vi "Get Connection from Statement.vi"(8 "error in (no error)":errorcluster, 11 "SQL Statement In":refnum<class "SQL Statement.lvclass">) -> (0 "error out":errorcluster, 2 "Connection out":refnum<class "Connection.lvclass">, 3 "SQL Statement Out":refnum<class "SQL Statement.lvclass">)   [LabVIEW 2023, in "SQLiteSupport.lvlib" / "SQL Statement.lvclass"]
uses:
  SQL Statement.lvclass
  SQL Connection/Connection.lvclass
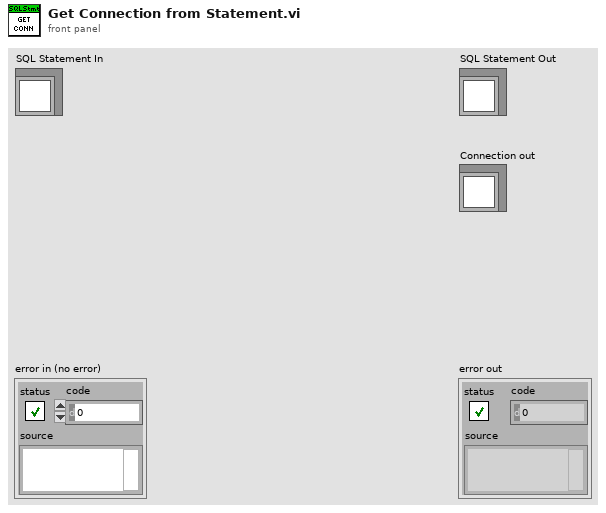
[diagram p1: front panel]
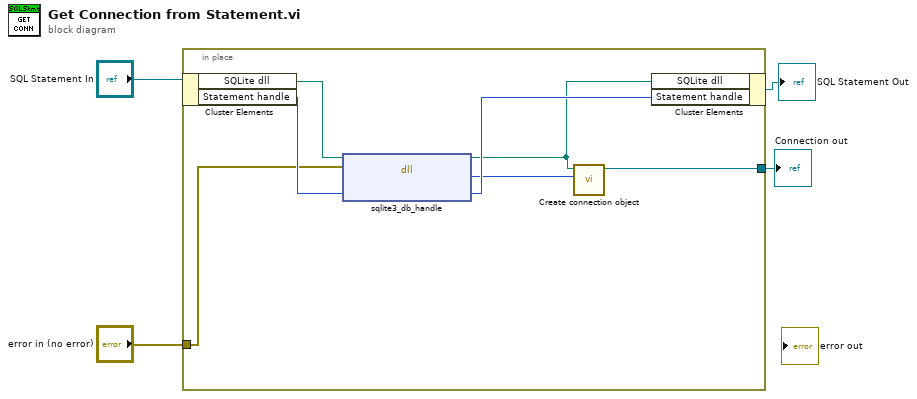
[diagram p0: block diagram]
diagram:
  n1 = in-place {
    in-place-border: "error in (no error)" -> [w8]
    in-place-border: [w5] -> w1
    n2 = in-place-cluster #1("SQL Statement In") -> ("SQLite dll"=w9:path, "Statement handle"=w10:u64)
    n3 = dll-call lib="C:/LabVIEW_JDP/Support/SQLite/SQL Connection/sqlite3.dll" fn="sqlite3_db_handle"(path in=w9, error in=w8, "stmt handle"=w10) -> (path out=w7:path, "db handle"=w6:u64, "stmt handle"=w11:u64)  [unwired: 1 in, 1 out]
    n4 = call "Create connection object.vi"("db handle"=w6, "SQLite dll"=w7) -> ("Connection out"=w5:refnum<class "Connection.lvclass">)  [unwired: 8 in, 1 out]
    n5 = in-place-cluster #1("SQLite dll"=w7, "Statement handle"=w11) -> (→"SQL Statement Out":refnum<class "SQL Statement.lvclass">)
  }
  "Connection out" <- w1
